vi "mainFPGA.vi"() -> ()   [LabVIEW 2021]
uses:
  <vilib>/rvi/Emulation/niFpgaGetClockAttributes.vi
  <vilib>/rvi/Emulation/niFpgaSctlEmulationGetInTimedLoop.vi
  <vilib>/rvi/Emulation/niFpgaEmulationReportErrorSimple.vi
  <vilib>/rvi/eio/common/nirviEmuTemplateMethod_errors.vi
  <vilib>/rvi/Emulation/niFpgaCriticalErrorInLSC.vi
  <vilib>/eio/EIONode/EIONode.xnode
panel:
  out "booleanInputsToIntegerOutput":u8
  in  "isSimulatorMode":bool
  in  "LED3":bool
  in  "LED2":bool
  in  "LED1":bool
  in  "LED0":bool
  in  "options":i16
  in  "integerToBoolArray":u8
  in  "integerInputs":u8
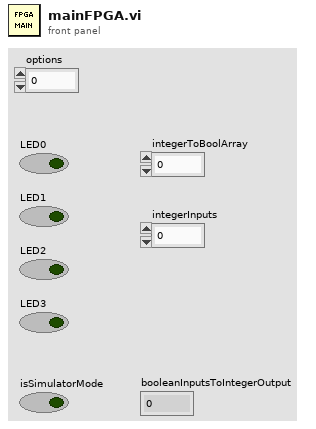
[diagram p1: front panel]
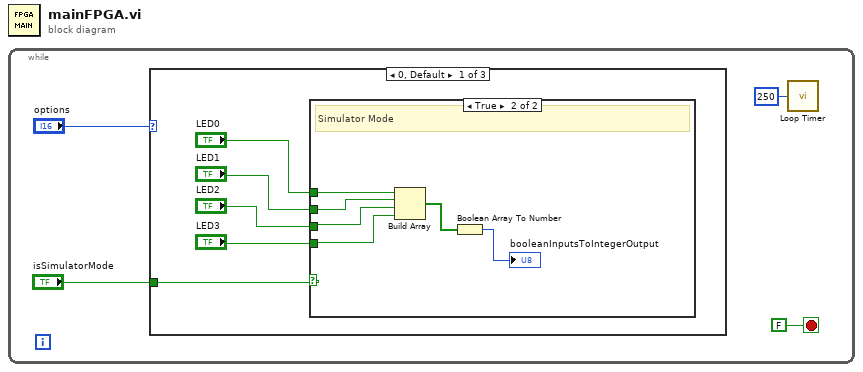
[diagram p0: block diagram]
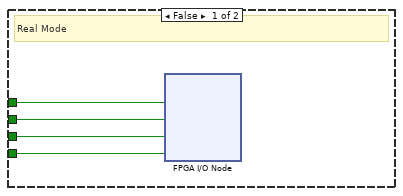
[diagram p2: hidden frame]
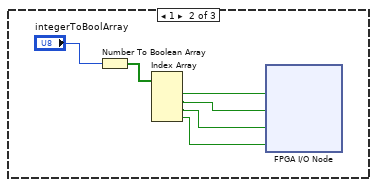
[diagram p3: hidden frame]
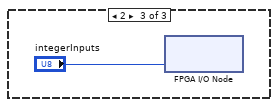
[diagram p4: hidden frame]
diagram:
  n1 = while {
    stop <- FALSE stop-if-true
    n2 = case shown="0, Default" "options" {
      tunnel: "isSimulatorMode" -> [w5 _ _]
      frame 0, Default {
        n3 = case shown="True" w5 {
          tunnel: "LED0" -> [w13 w19]
          tunnel: "LED1" -> [w12 w18]
          tunnel: "LED2" -> [w11 w17]
          tunnel: "LED3" -> [w10 w16]
          frame False {
            # "Real Mode"
            n4 = xnode "FPGA I/O Node"("LED0"=w13, "LED1"=w12, "LED2"=w11, "LED3"=w10) -> ()  [unwired: 4 in, 4 out]
          }
          frame True {
            # "Simulator Mode"
            n5 = Build Array "Build Array"(w19, w18, w17, w16) -> (w14:bool[])
            n6 = Boolean Array To Number(Boolean array=w14) -> (number=→"booleanInputsToIntegerOutput":u8)
          }
        }
      }
      frame 1 {
        n7 = Number To Boolean Array(number="integerToBoolArray") -> (Boolean array=w25:bool[])
        n8 = Index Array(array=w25) -> (element #1=w23:bool, element #2=w22:bool, element #3=w21:bool, element #4=w20:bool)  [unwired: 4 in]
        n9 = xnode "FPGA I/O Node"("LED0"=w23, "LED1"=w22, "LED2"=w21, "LED3"=w20) -> ()  [unwired: 4 in, 4 out]
      }
      frame 2 {
        n10 = xnode "FPGA I/O Node"("LED3:0"="integerInputs") -> ()  [unwired: 1 in, 1 out]
      }
    }
    n11 = call "Loop Timer"("Count(mSec)"=u32 250) -> ()  [unwired: 1 out]
  }
